vi "GVZwangsMPVPos_ECD.vi"() -> ()   [LabVIEW 2017]
panel:
  out "ZwangsMPV!":i32
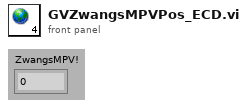
[diagram p1: front panel]
diagram:
